vi "Render Children.vi"(6 "Loader":refnum<class "Loader.lvclass">, 8 "Error In":errorcluster, 10 "Children":refnum<class "Node.lvclass">[](array[class]), 11 "Context In":refnum<class "Context.lvclass">) -> (0 "Error Out":errorcluster, 2 "Output":string, 3 "Context Out":refnum<class "Context.lvclass">)   [LabVIEW 2018, in "Toolkit.lvlib"]
uses:
  Toolkit.lvlib
  Context/Context/Context.lvclass
  Nodes/Node/Node.lvclass
  Loaders/Loader/Loader.lvclass
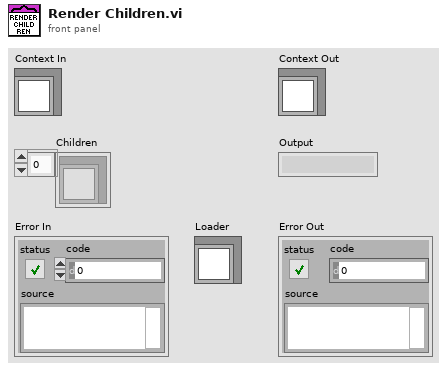
[diagram p1: front panel]
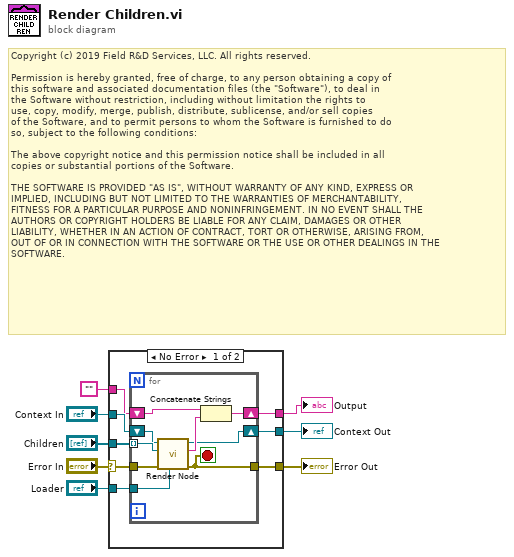
[diagram p0: block diagram]
diagram:
  # "Copyright (c) 2019 Field R&D Services, LLC. All rights reserved.\n\nPermission is hereby granted, free of charge, to any person obtaining a copy of\nthis software and associated documentation files (the \"Software\"), to deal in\nthe Software without restriction, including without limitation the rights to\nuse, copy, modify, merge, publish, distribute, sublicense, and/or sell copies\nof the Software, and to permit persons to whom the Software is furnished to do\nso, subject to the following conditions:\n\nThe above copyright notice and this permission notice shall be included in all\ncopies or substantial portions of the Software.\n\nTHE SOFTWARE IS PROVIDED \"AS IS\", WITHOUT WARRANTY OF ANY KIND, EXPRESS OR\nIMPLIED, INCLUDING BUT NOT LIMITED TO THE WARRANTIES OF MERCHANTABILITY,\nFITNESS FOR A PARTICULAR PURPOSE AND NONINFRINGEMENT. IN NO EVENT SHALL THE\nAUTHORS OR COPYRIGHT HOLDERS BE LIABLE FOR ANY CLAIM, DAMAGES OR OTHER\nLIABILITY, WHETHER IN AN ACTION OF CONTRACT, TORT OR OTHERWISE, ARISING FROM,\nOUT OF OR IN CONNECTION WITH THE SOFTWARE OR THE USE OR OTHER DEALINGS IN THE\nSOFTWARE."
  n1 = case shown="No Error" "Error In" {
    selector: "Error In" -> [w10 w26]
    tunnel: [w16 w28] -> w8
    tunnel: [w15 w26] -> w7
    tunnel: [w14 w27] -> w6
    tunnel: "Context In" -> [w13 w27]
    tunnel: "Children" -> [w12 _]
    tunnel: "" -> [w11 w28]
    tunnel: "Loader" -> [w9 _]
    frame No Error {
      n2 = for {
        tunnel: w10 -> [w18]
        tunnel: w12 -> [w23] mode=indexing
        tunnel: [w19] -> w15
        shift-right: [w24] -> w16
        shift-left: w11 -> [w25]
        shift-right: [w20] -> w14
        shift-left: w13 -> [w22]
        tunnel: w9 -> [w17]
        stop <- w19 stop-if-true
        n3 = call "Render Node.vi"("Loader"=w17, "Error In"=w18, "Node"=w23, "Context In"=w22) -> ("Error Out"=w19:errorcluster, "Output"=w21:string, "Context Out"=w20:refnum<class "Context.lvclass">)  [unwired: 5 in]
        n4 = Concatenate Strings(w25, w21) -> (w24:string)
      }
    }
    frame Error {
    }
  }
  "Output" <- w8
  "Error Out" <- w7
  "Context Out" <- w6
